vi "Trig OP Setup-Parser.vi"(0 "Triggers output setup to save":T4=[{"Name"="", "Output?"=FALSE, "Output terminal"="/PXI1Slot6/PFI0", "PXI backplane line"="/PXI1Slot6/PXI_Trig0", "Pulse width (us)"=20}, {"Name"="", "Output?"=FALSE, "Output terminal"="/PXI1Slot6/PFI0", "PXI backplane line"="/PXI1Slot6/PXI_Trig0", "Pulse width (us)"=20}, {"Name"="", "Output?"=FALSE, "Output terminal"="/PXI1Slot6/PFI0", "PXI backplane line"="/PXI1Slot6/PXI_Trig0", "Pulse width (us)"=20}, {"Name"="", "Output?"=FALSE, "Output terminal"="/PXI1Slot6/PFI0", "PXI backplane line"="/PXI1Slot6/PXI_Trig0", "Pulse width (us)"=20}, {"Name"="", "Output?"=FALSE, "Output terminal"="/PXI1Slot6/PFI0", "PXI backplane line"="/PXI1Slot6/PXI_Trig0", "Pulse width (us)"=20}, {"Name"="", "Output?"=FALSE, "Output terminal"="/PXI1Slot6/PFI0", "PXI backplane line"="/PXI1Slot6/PXI_Trig0", "Pulse width (us)"=20}] {"Pulse width (us)" min=10 max=5000 step=1 format="%.0fµs"}, 3 "General trigger settings":T1={"Trigger 1 function"=enum."Encoder trigger", "Triggers loop clock (MHz)"=80.0} {"Triggers loop clock (MHz)" format="%#_13g"}) -> (16 "Keys setup.Strings":T6=[{"key"="Control FPGA.MAC address", "Save?"=TRUE, "Default"="AABBCCDDEEFF"}, {"key"="DAQ FPGA.Target", "Save?"=TRUE, "Default"="RIO0"}, {"key"="XY Stage.COM port", "Save?"=TRUE, "Default"="COM7"}, {"key"="DAQmx Chan.Pockels Control", "Save?"=TRUE, "Default"=""}, {"key"="DAQmx Chan.Hard Shutter", "Save?"=TRUE, "Default"=""}, {"key"="DAQmx Chan.PMT 1", "Save?"=TRUE, "Default"=""}, {"key"="DAQmx Chan.PMT 2", "Save?"=TRUE, "Default"=""}, {"key"="DAQmx Chan.Encoder Trigger", "Save?"=TRUE, "Default"=""}, {"key"="DAQmx Chan.Optional Trigger 1", "Save?"=TRUE, "Default"=""}, {"key"="DAQmx Chan.Optional Trigger 2", "Save?"=TRUE, "Default"=""}, {"key"="DAQmx Chan.Optional Trigger 3", "Save?"=TRUE, "Default"=""}], 17 "Values.Strings":string[](array[string]), 18 "Keys setup.DBL":T3, 19 "Values.DBL":dbl[](array[numeric]))   [LabVIEW 2020]
uses:
  Typedefs/Ini file interface (String).ctl
  Peripherals Control/Triggers/Typedefs/Triggers output setup.ctl
  Peripherals Control/Triggers/Typedefs/Trigger setup element cluster.ctl
  Typedefs/Ini file interface (DBL).ctl
  Peripherals Control/Triggers/Typedefs/General trigger settings cluster.ctl
  Typedefs/Trigger 1 selector enum.ctl
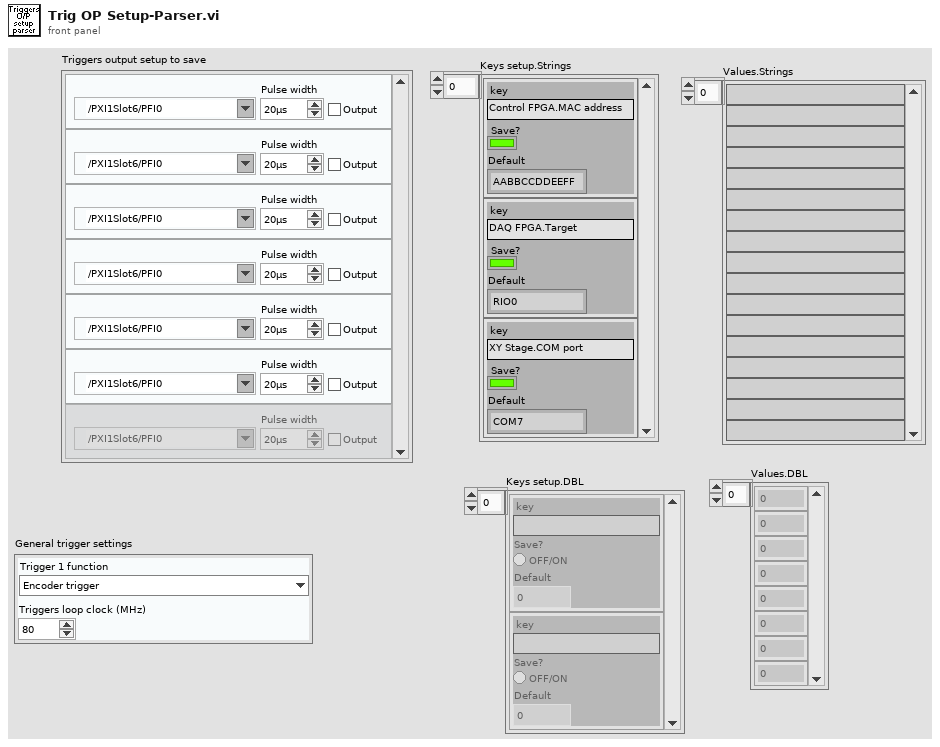
[diagram p1: front panel]
types:
  T1 = typedef "General trigger settings cluster.ctl" = cluster{"Trigger 1 function":T2, "Triggers loop clock (MHz)":dbl}
  T2 = typedef "Trigger 1 selector enum.ctl" = enum16{"Encoder trigger", "Line trigger", "Control system's ref frame acknowledgement"}
  T3 = typedef "Ini file interface (DBL).ctl" = cluster{"key":string, "Save?":bool, "Default":dbl}[]
  T4 = typedef "Triggers output setup.ctl" = T5[]
  T5 = typedef "Trigger setup element cluster.ctl" = cluster{"Name":string, "Output?":bool, "Output terminal":tag, "PXI backplane line":tag, "Pulse width (us)":u16}
  T6 = typedef "Ini file interface (String).ctl" = cluster{"key":string, "Save?":bool, "Default":string}[]
  T7 = cluster{"key":string, "Save?":bool, "Default":string}[]
  T8 = cluster{"Name":string, "Output":bool, "Output terminal":tag, "PXI backplane line":tag, "Pulse width":u16}[]
  T9 = cluster{"key":string, "Save?":bool, "Default":string}
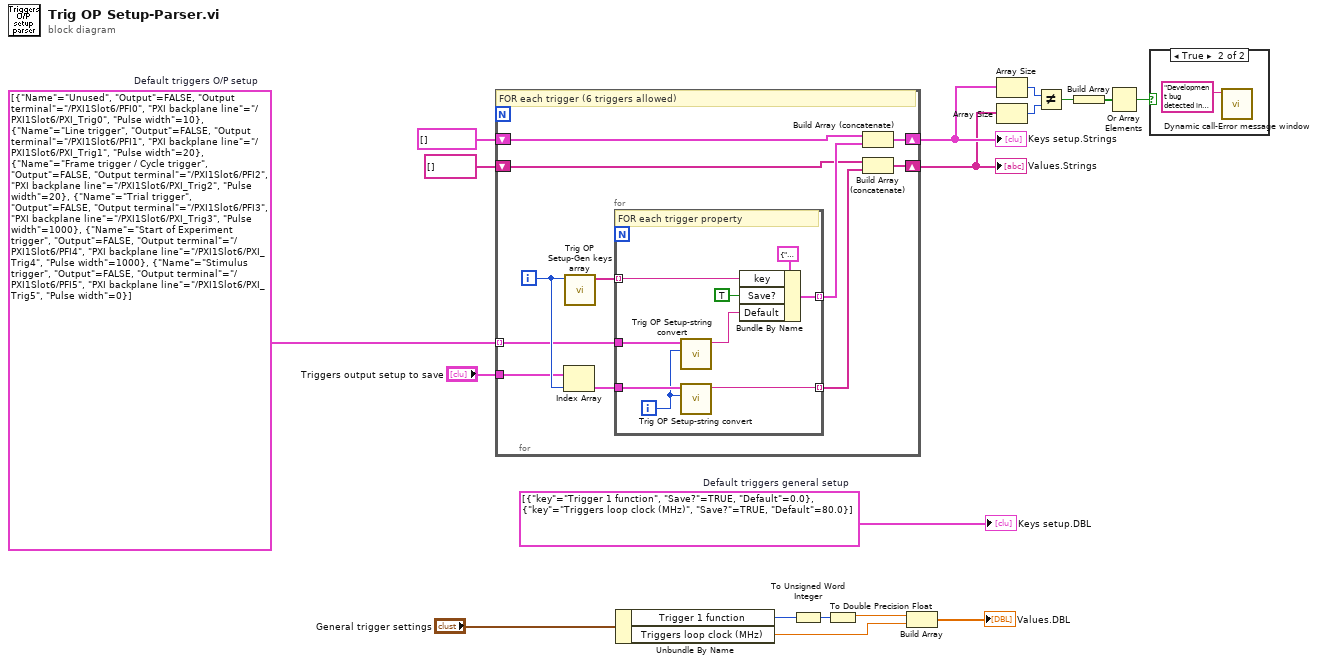
[diagram p0: block diagram]
diagram:
  w7 = T3 [{"key"="Trigger 1 function", "Save?"=TRUE, "Default"=0.0}, {"key"="Triggers loop clock (MHz)", "Save?"=TRUE, "Default"=80.0}]  # Default triggers general setup
  w8 = T8 [{"Name"="Unused", "Output"=FALSE, "Output terminal"="/PXI1Slot6/PFI0", "PXI backplane line"="/PXI1Slot6/PXI_Trig0", "Pulse width"=10}, {"Name"="Line trigger", "Output"=FALSE, "Output terminal"="/PXI1Slot6/PFI1", "PXI backplane line"="/PXI1Slot6/PXI_Trig1", "Pulse width"=20}, {"Name"="Frame trigger / Cycle trigger", "Output"=FALSE, "Output terminal"="/PXI1Slot6/PFI2", "PXI backplane line"="/PXI1Slot6/PXI_Trig2", "Pulse width"=20}, {"Name"="Trial trigger", "Output"=FALSE, "Output terminal"="/PXI1Slot6/PFI3", "PXI backplane line"="/PXI1Slot6/PXI_Trig3", "Pulse width"=1000}, {"Name"="Start of Experiment trigger", "Output"=FALSE, "Output terminal"="/PXI1Slot6/PFI4", "PXI backplane line"="/PXI1Slot6/PXI_Trig4", "Pulse width"=1000}, {"Name"="Stimulus trigger", "Output"=FALSE, "Output terminal"="/PXI1Slot6/PFI5", "PXI backplane line"="/PXI1Slot6/PXI_Trig5", "Pulse width"=0}]  # Default triggers O/P setup
  n1 = for {
    tunnel: "Triggers output setup to save" -> [w20]
    shift-right: [w26] -> w10
    shift-left: T7 [] -> [w25]
    shift-right: [w23] -> w9
    shift-left: string[] [] -> [w22]
    tunnel: w8 -> [w21] mode=indexing
    i -> [w28]
    # "FOR each trigger (6 triggers allowed)"
    n2 = Index Array(array=w20, index=w28) -> (element=w19:T5)
    n3 = call "Trig OP Setup-Gen keys array.vi"("Trigger index (FOR loop index)"=w28) -> ("Keys array for each trigger"=w29:string[])  [unwired: 10 in]
    n4 = for {
      tunnel: w29 -> [w38] mode=indexing
      tunnel: w21 -> [w37]
      tunnel: [w33] -> w27 mode=indexing
      tunnel: w19 -> [w32]
      tunnel: [w31] -> w24 mode=indexing
      i -> [w30]
      # "FOR each trigger property"
      n5 = call "Trig OP Setup-string convert.vi"("FOR loop index"=w30, "Trigger setup element"=w37) -> ("String"=w34:string)  [unwired: 9 in]
      n6 = call "Trig OP Setup-string convert.vi"("FOR loop index"=w30, "Trigger setup element"=w32) -> ("String"=w31:string)  [unwired: 9 in]
      n7 = Bundle By Name(cluster=T9 {"key"="", "Save?"=TRUE, "Default"=""}, "key"=w38, "Save?"=TRUE, "Default"=w34) -> (w33:T9)
    }
    n8 = Build Array (concatenate)(w25, w27) -> (w26:T7)
    n9 = Build Array (concatenate)(w22, w24) -> (w23:string[])
  }
  "Keys setup.Strings" <- w10
  "Values.Strings" <- w9
  n10 = Unbundle By Name("General trigger settings") -> ("Trigger 1 function"=w5:T2, "Triggers loop clock (MHz)"=w2:dbl)
  n11 = To Unsigned Word Integer(number=w5) -> (unsigned 16bit integer=w4:u16)
  n12 = To Double Precision Float(number=w4) -> (double precision float=w3:dbl)
  n13 = Build Array(w3, w2) -> (→"Values.DBL":dbl[])
  n14 = Array Size(array=w10) -> (size(s)=w15:i32)
  n15 = Array Size(array=w9) -> (size(s)=w14:i32)
  n16 = Not Equal?(x=w15, y=w14) -> (x != y?=w11:bool)
  n17 = Build Array(w11) -> (w13:bool[])
  n18 = Or Array Elements(Boolean array=w13) -> (logical OR=w12:bool)
  n19 = case shown="True" w12 {
    frame False {
    }
    frame True {
      n20 = call "Dynamic call-Error message window.vi"("Error Message"="Development bug detected in the \"Trig OP Setup-Parser.vi\".\nPlease correct the set up in this VI.") -> ()  [unwired: 10 in, 1 out]
    }
  }
  "Keys setup.DBL" <- w7
